vi "剖面数据模拟器.vi"() -> ()   [LabVIEW 2016]
uses:
  <vilib>/Utility/miscctls.llb/LVPointTypeDef.ctl
panel:
  in  "Password":string
  out "缓存":T1[](array[typedef])
  out "data":T1
  in  "Tabe Name":string
  in  "错误输入（无错误）":errorcluster
  out "错误输出":errorcluster
  in  "数据库类型":T2
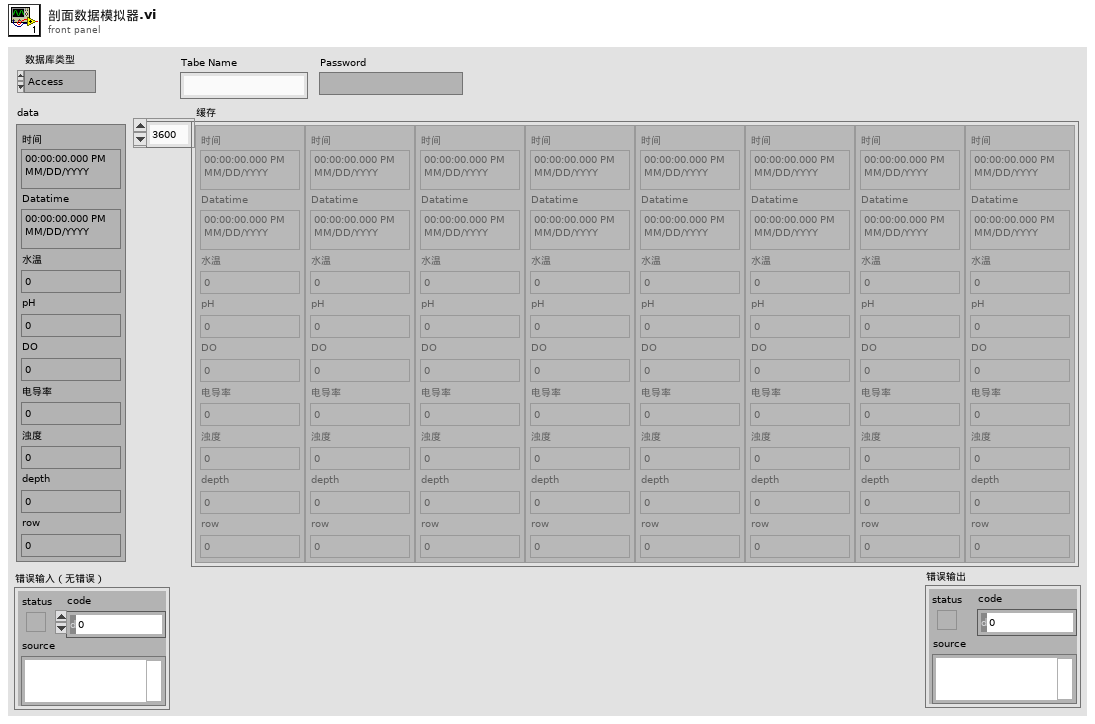
[diagram p1: front panel]
types:
  T1 = typedef "剖面数据字段定义.ctl" = cluster{"时间":timestamp, "Datatime":timestamp, "水温":sgl, "pH":sgl, "DO":sgl, "电导率":sgl, "浊度":sgl, "depth":sgl, "row":u32}
  T2 = typedef "数据库类型.ctl" = enum16{"Access", "SQLite"}
  T3 = typedef "LVPointTypeDef.ctl" = cluster{"Horizontal":i16, "Vertical":i16}
  T4 = typedef "LVDateTimeRec.ctl" = cluster{"秒数的小数部分":dbl, "秒":i32, "分":i32, "时":i32, "日":i32, "月":i32, "年":i32, "天数（周）":i32, "天数（年）":i32, "DST":i32}
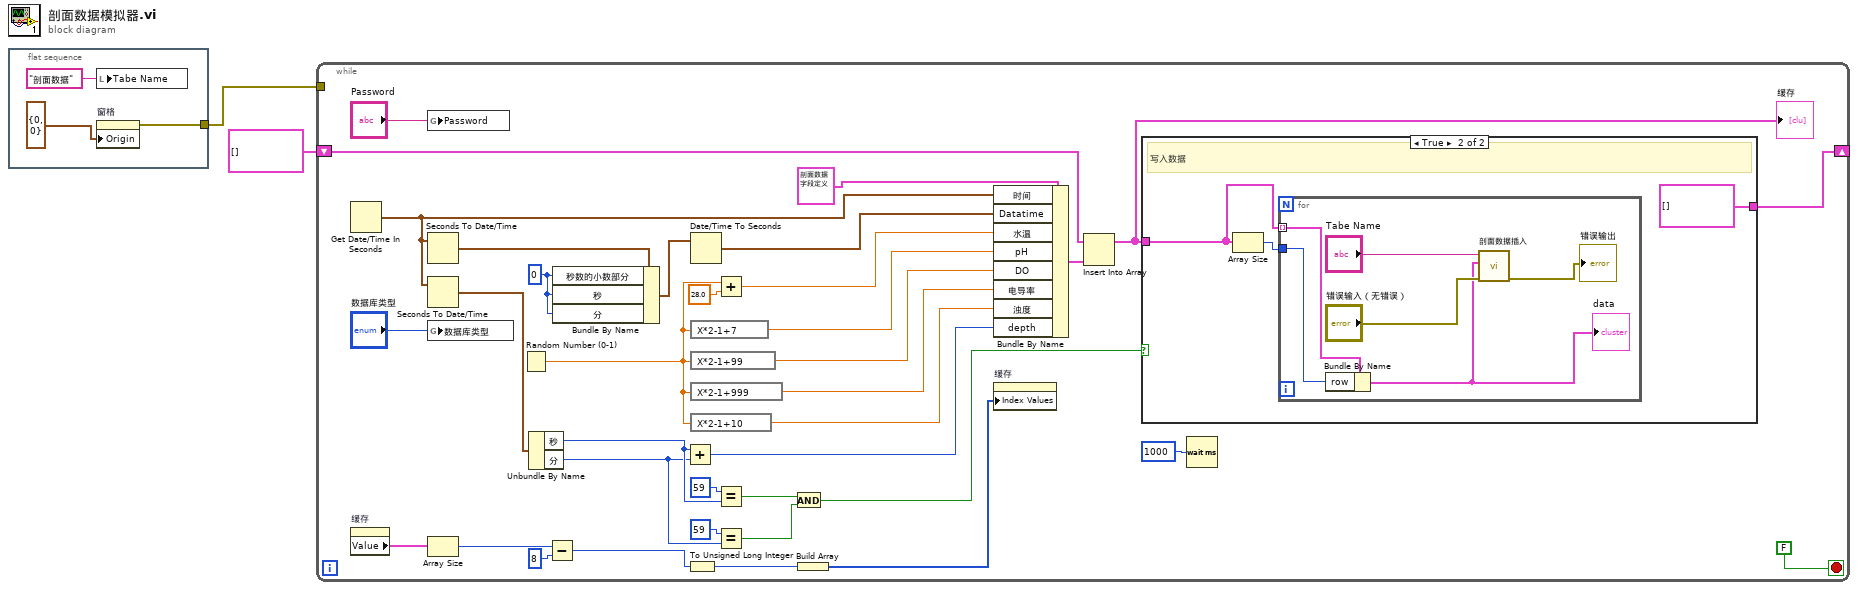
[diagram p0: block diagram]
diagram:
  n1 = flat-sequence {
    tunnel: [w4] -> w2
    frame #0 {
      n2 = local write "Tabe Name"("剖面数据" ("Tabe Name")) -> ()
      n3 = property on="窗格" class="Pane"("Origin"=T3 {"Horizontal"=0, "Vertical"=0} ("原点")) -> (error out=w4:errorcluster)  [unwired: 2 in, 1 out]
    }
  }
  n4 = while {
    tunnel: w2 -> [_]
    shift-right: [w19] -> _
    shift-left: T1[] [] -> [w35]
    stop <- FALSE stop-if-true
    w30 = 0 ("秒")
    n5 = Get Date/Time In Seconds() -> (seconds since 1Jan1904=w27:timestamp)
    n6 = property on="缓存" class="Arr (strict)"() -> ("Value"=w15:T1[])  [unwired: 2 in, 2 out]
    n7 = global write "外部调用接口全局变量.vi" "Password"("Password") -> ()
    n8 = Seconds To Date/Time(time stamp (now)=w27) -> (date time rec=w31:T4)  [unwired: 1 in]
    n9 = Seconds To Date/Time(time stamp (now)=w27) -> (date time rec=w32:T4)  [unwired: 1 in]
    n10 = global write "外部调用接口全局变量.vi" "数据库类型"("数据库类型") -> ()
    n11 = Array Size(array=w15) -> (size(s)=w14:i32)
    n12 = Random Number (0-1)() -> (number: 0 to 1=w21:dbl)
    n13 = Unbundle By Name(w32) -> ("秒"=w18:i32, "分"=w17:i32)
    n14 = Subtract(x=w14, y=8) -> (x-y=w12:i32)
    n15 = Bundle By Name(cluster=w31, "秒数的小数部分"=w30, "秒"=w30, "分"=w30) -> (w28:T4)
    n16 = Add(x=w18, y=w17) -> (x+y=w16:i32)
    n17 = To Unsigned Long Integer(number=w12) -> (unsigned 32bit integer=w11:u32)
    n18 = Date/Time To Seconds(2:w28) -> (0:w29:timestamp)  [unwired: 1 in]
    n19 = expression code="X*2-1+7"(w21) -> (w24:dbl)
    n20 = expression code="X*2-1+99"(w21) -> (w23:dbl)
    n21 = expression code="X*2-1+999"(w21) -> (w22:dbl)
    n22 = expression code="X*2-1+10"(w21) -> (w20:dbl)
    n23 = Add(x=w21, y=28.0) -> (x+y=w25:dbl)
    n24 = Equal?(x=59, y=w18) -> (x = y?=w39:bool)
    n25 = Equal?(x=59, y=w17) -> (x = y?=w38:bool)
    n26 = And(x=w39, y=w38) -> (x .and. y?=w37:bool)
    n27 = Build Array(w11) -> (w10:u32[])
    n28 = Bundle By Name(cluster=T1 {"时间"=timestamp(0 s since 1904-01-01), "Datatime"=timestamp(0 s since 1904-01-01), "水温"=0.0, "pH"=0.0, "DO"=0.0, "电导率"=0.0, "浊度"=0.0, "depth"=0.0, "row"=0} ("data"), "时间"=w27, "Datatime"=w29, "水温"=w25, "pH"=w24, "DO"=w23, "电导率"=w22, "浊度"=w20, "depth"=w16) -> (w33:T1)
    n29 = property on="缓存" class="Arr (strict)"("Index Values"=w10) -> ()  [unwired: 2 in, 2 out]
    n30 = Insert Into Array(array=w35, new element=w33) -> (w36:T1[])  [unwired: 1 in]
    "缓存" <- w36
    n31 = case shown="True" w37 {
      tunnel: w36 -> [w42 w44]
      tunnel: [w42 T1[] []] -> w19
      frame False {
      }
      frame True {
        # "写入数据"
        n32 = Array Size(array=w44) -> (size(s)=w43:i32)
        n33 = for {
          tunnel: w44 -> [w48] mode=indexing
          tunnel: w43 -> [w47]
          n34 = Bundle By Name(cluster=w48, "row"=w47) -> (w46:T1)
          "data" <- w46
          n35 = call "剖面数据插入.vi"("Tabe Name"="Tabe Name", "data"=w46, "错误输入（无错误）"="错误输入（无错误）") -> ("错误输出"=→"错误输出":errorcluster)  [unwired: 7 in]
        }
      }
    }
    n36 = Wait (ms)(milliseconds to wait=u32 1000 ("等待时间（毫秒）")) -> ()  [unwired: 1 out]
  }
